vi "Table_InitialTableValues.vi"(8 "error in":errorcluster, 11 "Channel Selection":T1[](array[typedef])) -> (0 "error out":errorcluster, 3 "Table Values":string[][](array[string]))   [LabVIEW 2012, in "TableSupportLib.lvlib"]
uses:
  TableSupportLib.lvlib
  Table_ChannelInfoCluster.ctl
  Table_Globals.vi
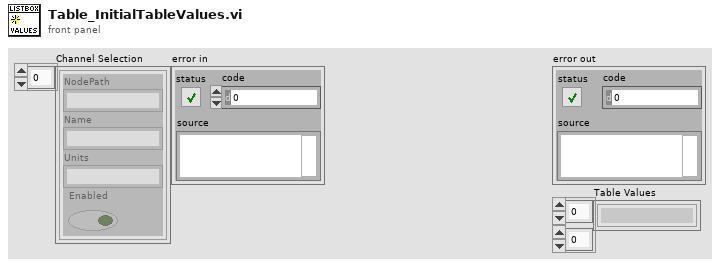
[diagram p1: front panel]
types:
  T1 = typedef "TableSupportLib.lvlib/Table_ChannelInfoCluster.ctl" = cluster{"NodePath":string, "Name":string, "Units":string, "Enabled":bool}
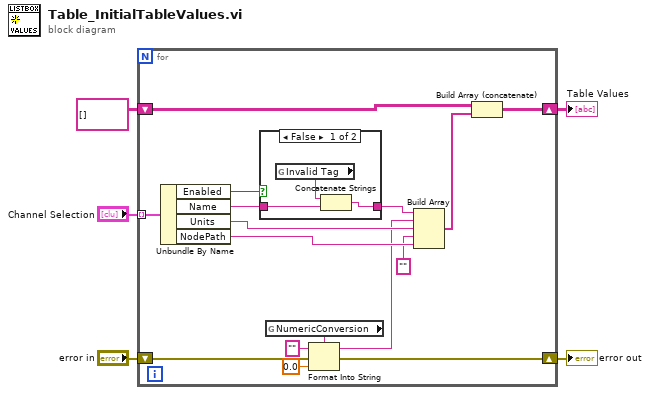
[diagram p0: block diagram]
diagram:
  n1 = for {
    tunnel: "Channel Selection" -> [w21] mode=indexing
    shift-right: [w19] -> w1
    shift-left: string[][] [] -> [w18]
    shift-right: [w16] -> w3
    shift-left: "error in" -> [w17]
    n2 = Unbundle By Name(w21) -> ("Enabled"=w7:bool, "Name"=w9:string, "Units"=w20:string, "NodePath"=w15:string)
    n3 = case shown="False" w7 {
      tunnel: w9 -> [w24 w25]
      tunnel: [w23 w25] -> w8
      frame False {
        n4 = global read "Table_Globals.vi" "Invalid Tag"() -> (w22:string)
        n5 = Concatenate Strings(w22, w24) -> (w23:string)
      }
      frame True {
      }
    }
    n6 = global read "Table_Globals.vi" "NumericConversion"() -> (w11:string)
    n7 = Format Into String(format string=w11, initial string="", error in=w17, 0.0 ("input 1")) -> (resulting string=w12:string, error out=w16:errorcluster)
    n8 = Build Array(w8, w12, w20, "", w15) -> (w10:string[])
    n9 = Build Array (concatenate)(w18, w10) -> (w19:string[][])
  }
  "error out" <- w3
  "Table Values" <- w1
